vi "VtoPerc.vi"(1 "Volt":dbl) -> (0 "Perc":dbl)   [LabVIEW 2016]
doc: "Подпрограмма предназначена для перевода считанного\nс DAQ напряжения в диапазоне 1-5В в технологические\n% в диапазоне 0-100"
panel:
  # "Подпрограмма предназначена для перевода считанного\nс DAQ напряжения в диапазоне 1-5В в технологические\n% в диапазоне 0-100"
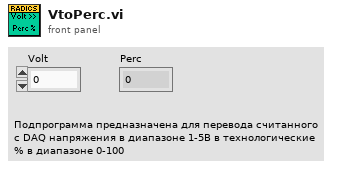
[diagram p1: front panel]
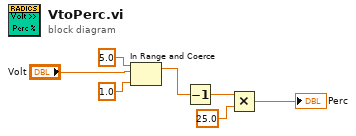
[diagram p0: block diagram]
diagram:
  n1 = In Range and Coerce(upper limit=5.0, x="Volt", lower limit=1.0) -> (coerced(x)=w5:dbl)  [unwired: 1 out]
  n2 = Decrement(x=w5) -> (x-1=w6:dbl)
  n3 = Multiply(x=w6, y=25.0) -> (x*y=→"Perc":dbl)
